vi "Format File Property.vi"(8 "错误输入":cluster{"状态":bool, "代码":i32, "源":string}, 9 "文件属性值":string, 10 "文件属性名称":string, 11 "字符串输入":string) -> (0 "错误输出":cluster{"状态":bool, "代码":i32, "源":string}, 3 "字符串输出":string)   [LabVIEW 2012]
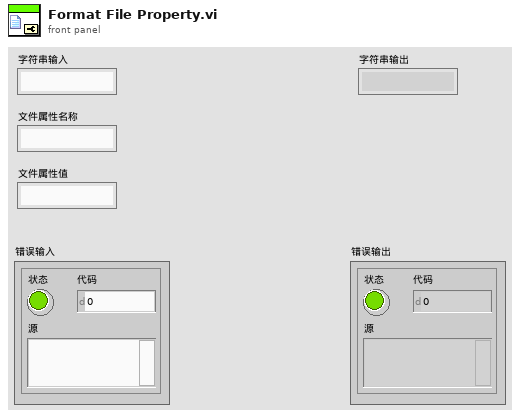
[diagram p1: front panel]
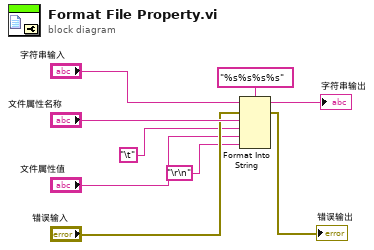
[diagram p0: block diagram]
diagram:
  n1 = Format Into String ("格式化写入字符串")(format string="%s%s%s%s" ("格式字符串"), initial string="字符串输入", error in="错误输入", "文件属性名称", "\t" ("制表符常量"), "文件属性值", "\r\n" ("行结束常量")) -> (resulting string=→"字符串输出":string, error out=→"错误输出":errorcluster)
